vi "Read Container Bounds.vi"(8 "error in (no error)":errorcluster, 11 "ActiveX Control in":refnum<class "ActiveXContainer.lvclass">) -> (0 "error out":errorcluster, 2 "Bounds":T1, 3 "ActiveX Control out":refnum<class "ActiveXContainer.lvclass">)   [LabVIEW 2020, in "WebView2 QControl.lvlib" / "ActiveXContainer.lvclass"]
uses:
  ActiveXContainer.lvclass
  ActiveXContainer.lvclass/ActiveXContainer.ctl
  <vilib>/Utility/miscctls.llb/LVBoundsTypeDef.ctl
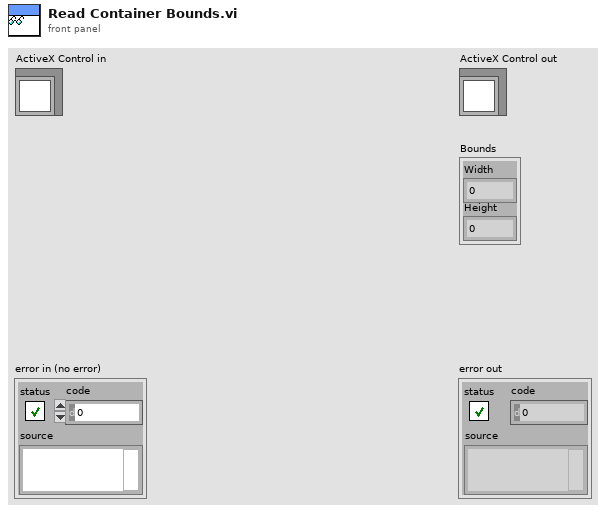
[diagram p1: front panel]
types:
  T1 = typedef "LVBoundsTypeDef.ctl" = cluster{"Width":u32, "Height":u32}
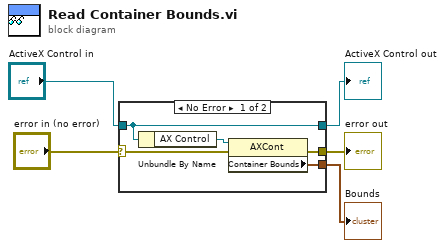
[diagram p0: block diagram]
diagram:
  n1 = case shown="No Error" "error in (no error)" {
    selector: "error in (no error)" -> [w10 w11]
    tunnel: [w8 w11] -> w4
    tunnel: [w9 w12] -> w2
    tunnel: "ActiveX Control in" -> [w9 w12]
    tunnel: [w6 _] -> w1
    frame No Error {
      n2 = Unbundle By Name(w9) -> ("AX Control"=w7:refnum<vi>)
      n3 = property class="AXCont"(reference=w7, error in=w10) -> (error out=w8:errorcluster, "Container Bounds"=w6:T1)  [unwired: 1 out]
    }
    frame Error {
    }
  }
  "error out" <- w4
  "ActiveX Control out" <- w2
  "Bounds" <- w1
